vi "invert_waveform_array.vi"(7 "Invert x":bool, 11 "x, y, z axis data":waveform(dbl)[](array[waveform])) -> (3 "inverted x waveform array":waveform(dbl)[](array[waveform]))   [LabVIEW 2020]
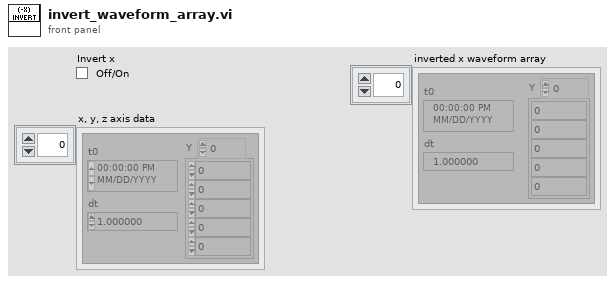
[diagram p1: front panel]
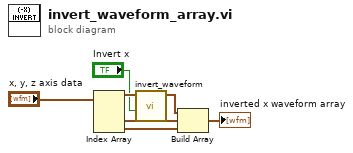
[diagram p0: block diagram]
diagram:
  n1 = Index Array(array="x, y, z axis data") -> (element #1=w3:waveform(dbl), element #2=w5:waveform(dbl), element #3=w6:waveform(dbl))  [unwired: 3 in]
  n2 = call "invert_waveform.vi"("invert"="Invert x", "waveform"=w3) -> ("output waveform"=w4:waveform(dbl))  [unwired: 9 in]
  n3 = Build Array(w4, w5, w6) -> (→"inverted x waveform array":waveform(dbl)[])
